vi "create swept sine.vi"(7 "invert scan direction":bool, 8 "sampling period [us] in":dbl=0.000833333333 format="%#_13g", 9 "duration [us]":dbl=340.0, 10 "bandwidth [MHz]":dbl=10.0, 11 "center freq [MHz]":dbl=105.0) -> (2 "sampling period [us] out":dbl=0.000833333333, 3 "waveform":dbl[](array[numeric]))   [LabVIEW 2024]
panel:
  out "Numeric":i32=120000
  out "x*y 4":dbl=100000000.0
  out "x*y 3":dbl=10000000.0
  out "x*y 2":dbl=9.999999999999999e-05
  out "x*y":dbl=9.999916662666699e-05
  out "Waveform Graph":dbl[](graph)
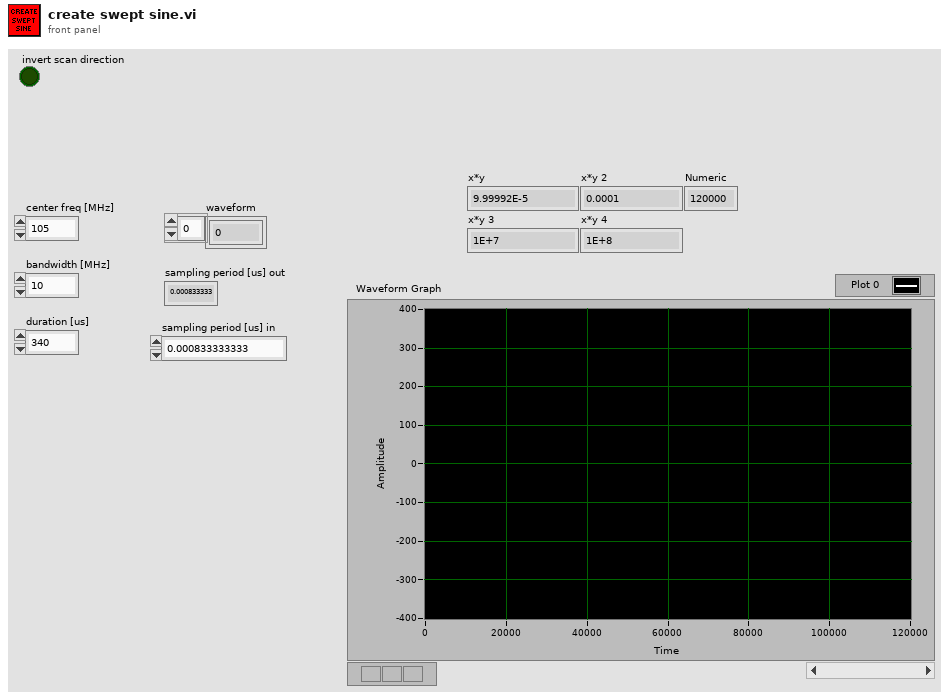
[diagram p1: front panel]
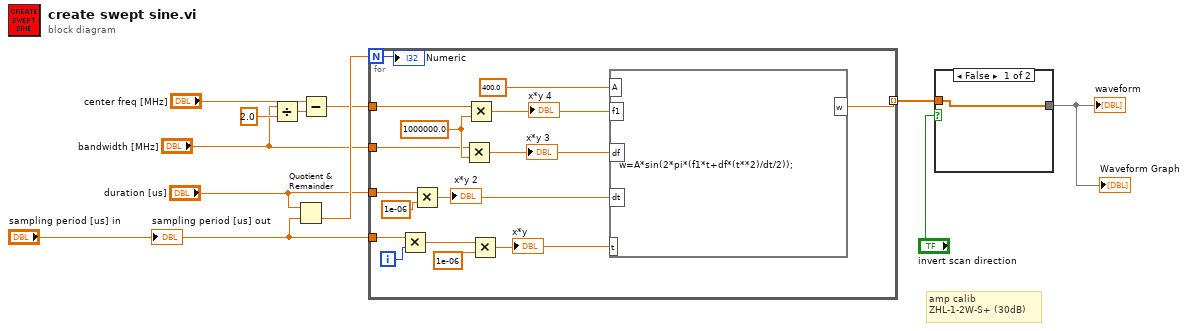
[diagram p0: block diagram]
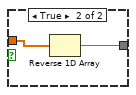
[diagram p2: hidden frame]
diagram:
  # "amp calib\nZHL-1-2W-S+ (30dB)"
  n1 = Divide(x="bandwidth [MHz]", y=2.0) -> (x/y=w11:dbl)
  n2 = Quotient & Remainder(x="duration [us]", y="sampling period [us] in") -> (floor(x/y)=w8:dbl)  [unwired: 1 out]
  n3 = Subtract(x="center freq [MHz]", y=w11) -> (x-y=w7:dbl)
  n4 = for {
    N: w8 -> [w12]
    tunnel: "sampling period [us] in" -> [w27]
    tunnel: w7 -> [w24]
    tunnel: "bandwidth [MHz]" -> [w22]
    tunnel: [w14] -> w2 mode=indexing
    tunnel: "duration [us]" -> [w13]
    i -> [w26]
    w23 = 1000000.0
    n5 = Multiply(x=w27, y=w26) -> (x*y=w15:dbl)
    n6 = Multiply(x=w13, y=1e-06) -> (x*y=w17:dbl)
    "x*y 2" <- w17
    n7 = Multiply(x=w22, y=w23) -> (x*y=w20:dbl)
    "x*y 3" <- w20
    n8 = Multiply(x=w24, y=w23) -> (x*y=w21:dbl)
    "x*y 4" <- w21
    n9 = Multiply(x=w15, y=1e-06) -> (x*y=w16:dbl)
    "x*y" <- w16
    n10 = formula code="w=A*sin(2*pi*(f1*t+df*(t**2)/dt/2));"("A"=400.0 ("input variable"), "f1"=w21, "df"=w20, "dt"=w17, "t"=w16) -> ("w"=w14:dbl)
    "Numeric" <- w12
  }
  n11 = case shown="False" "invert scan direction" {
    tunnel: w2 -> [w28 w30]
    tunnel: [w28 w29] -> w1
    frame False {
    }
    frame True {
      n12 = Reverse 1D Array(array=w30) -> (reversed array=w29:dbl[])
    }
  }
  "waveform" <- w1
  "Waveform Graph" <- w1
  "sampling period [us] out" <- "sampling period [us] in"
